vi "Channels.Inline.Reference Error Handler.vi"(8 "error in (no error)":errorcluster, 11 "pointer valid?":bool) -> (0 "error out":errorcluster)   [LabVIEW 2016, in "VeriStand Data.lvlib"]
doc: "Generates an error if a pointer is invalid."
uses:
  VeriStand Data.lvlib
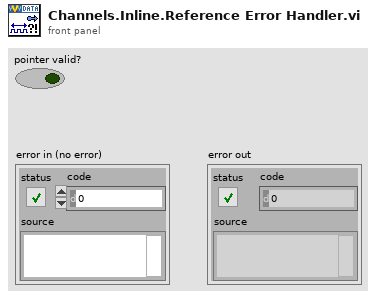
[diagram p1: front panel]
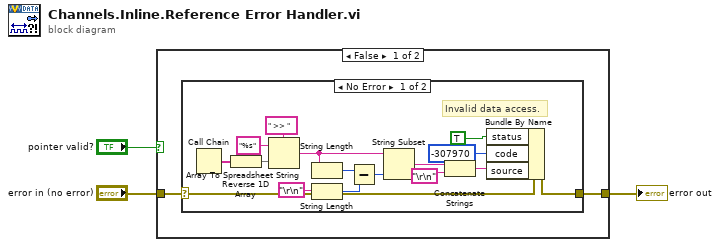
[diagram p0: block diagram]
diagram:
  n1 = case shown="False" "pointer valid?" {
    tunnel: "error in (no error)" -> [w5 w23]
    tunnel: [w4 w23] -> w2
    frame False {
      n2 = case shown="No Error" w5 {
        selector: w5 -> [w18 w22]
        tunnel: [w21 w22] -> w4
        frame No Error {
          # "Invalid data access."
          n3 = Call Chain() -> (call chain=w7:string[])
          n4 = Reverse 1D Array(array=w7) -> (reversed array=w14:string[])
          n5 = Array To Spreadsheet String(delimiter (Tab)=" >> ", array=w14, 3:"%s" ("format string")) -> (spreadsheet string=w15:string)
          n6 = String Length(string=w15) -> (length=w13:i32)
          n7 = String Length(string="\r\n") -> (length=w17:i32)
          n8 = Subtract(x=w13, y=w17) -> (x-y=w12:i32)
          n9 = String Subset(string=w15, length (rest)=w12) -> (substring=w8:string)  [unwired: 1 out]
          n10 = Concatenate Strings(w8, "\r\n") -> (w6:string)
          n11 = Bundle By Name(cluster=w18, "status"=TRUE, "code"=-307970, "source"=w6) -> (w21:errorcluster)
        }
        frame Error {
          # "Leave existing error."
        }
      }
    }
    frame True {
    }
  }
  "error out" <- w2
